vi "UpdateChannelsList.vi"(8 "error in (no error)":errorcluster, 10 "Channels":T1, 11 "ByteGSAPIBase in":refnum<class "ByteGSAPIBase.lvclass">) -> (0 "error out":errorcluster, 3 "ByteGSAPIBase out":refnum<class "ByteGSAPIBase.lvclass">)   [LabVIEW 2019, in "ByteGSWebAPI.lvlib" / "ByteGSAPIBase.lvclass"]
uses:
  ByteGSAPIBase.lvclass
  fields.ctl
  ByteGSAPIBase.lvclass/ByteGSAPIBase.ctl
  <vilib>/Bytelabs/ByteREST/ByteRESTClass/ByteRESTBase/RESTBase.lvclass
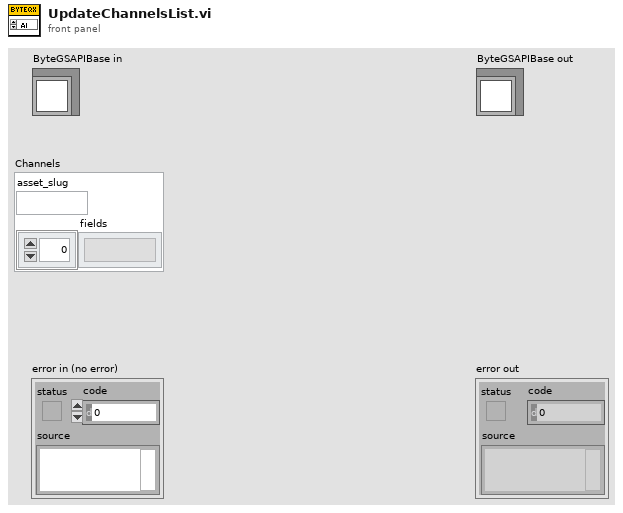
[diagram p1: front panel]
types:
  T1 = typedef "ByteGSWebAPI.lvlib/ByteGSAPIBase.lvclass/fields.ctl" = cluster{"asset_slug":string, "fields":string[]}
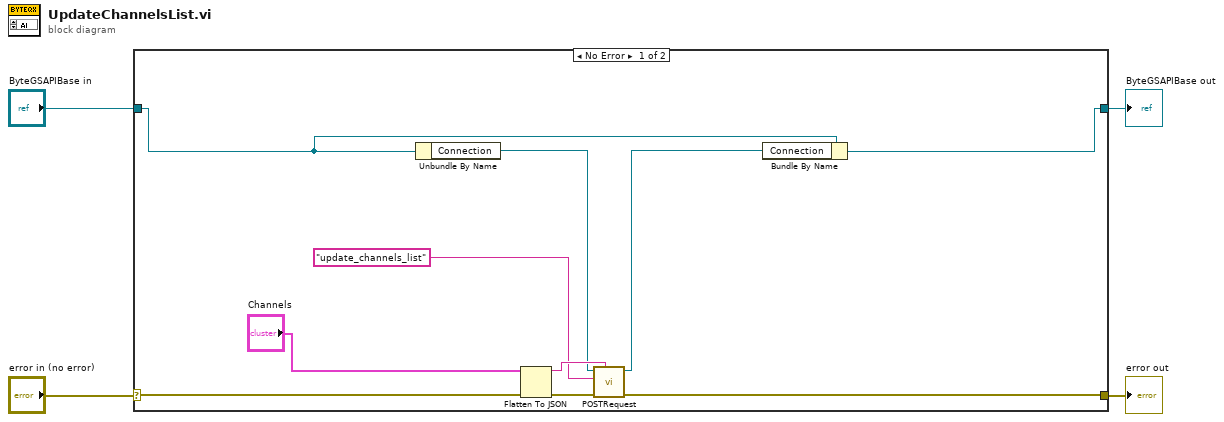
[diagram p0: block diagram]
diagram:
  n1 = case shown="No Error" "error in (no error)" {
    selector: "error in (no error)" -> [w9 w16]
    tunnel: [w8 w16] -> w3
    tunnel: [w5 w15] -> w1
    tunnel: "ByteGSAPIBase in" -> [w6 w15]
    frame No Error {
      n2 = Unbundle By Name(w6) -> ("Connection"=w12:refnum<class "RESTBase.lvclass">)
      n3 = Flatten To JSON(anything="Channels", error in (no error)=w9) -> (JSON string=w14:string, 11:w13:errorcluster)  [unwired: 1 in]
      n4 = call-dynamic "POSTRequest.vi"("Body in"=w14, "error in (no error)"=w13, "Request"="update_channels_list", "ByteRESTBase in"=w12) -> ("error out"=w8:errorcluster, "ByteRESTBase out"=w11:refnum<class "RESTBase.lvclass">)  [unwired: 4 in, 2 out]
      n5 = Bundle By Name(cluster=w6, "Connection"=w11) -> (w5:refnum<class "ByteGSAPIBase.lvclass">)
    }
    frame Error {
    }
  }
  "error out" <- w3
  "ByteGSAPIBase out" <- w1
